vi "L2.vi"() -> ()   [LabVIEW 2014]
panel:
  out "Boolean":bool
  in  "LIMITARE":bool
  out "Tank":dbl(slide) scale=0.0..10.0 scale format="%#_2g"
  in  "MAX":dbl(slide) scale=0.0..10.0
  in  "MIN":dbl(slide) scale=0.0..10.0
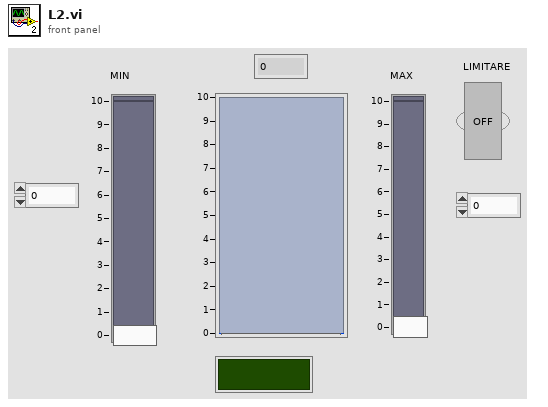
[diagram p1: front panel]
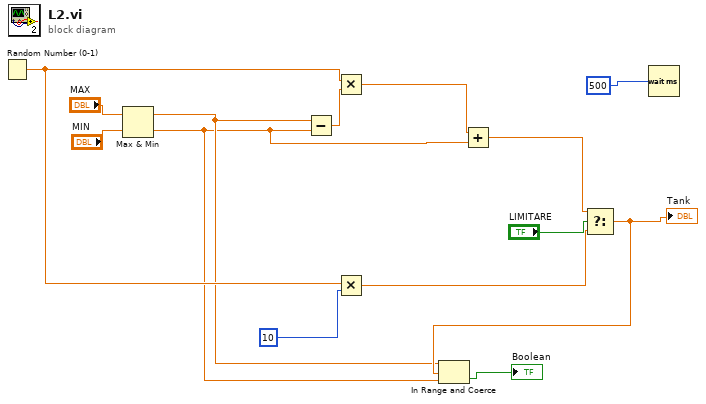
[diagram p0: block diagram]
diagram:
  n1 = Random Number (0-1)() -> (number: 0 to 1=w12:dbl)
  n2 = Max & Min(x="MAX", y="MIN") -> (max(x,y)=w2:dbl, min(x,y)=w1:dbl)
  n3 = Subtract(x=w2, y=w1) -> (x-y=w14:dbl)
  n4 = Multiply(x=w12, y=w14) -> (x*y=w13:dbl)
  n5 = Multiply(x=w12, y=10) -> (x*y=w8:dbl)
  n6 = Add(x=w13, y=w1) -> (x+y=w9:dbl)
  n7 = Select(t=w9, s="LIMITARE", f=w8) -> (s? t:f=w7:dbl)
  "Tank" <- w7
  n8 = In Range and Coerce(upper limit=w2, x=w7, lower limit=w1) -> (In Range?=→"Boolean":bool)  [unwired: 1 out]
  n9 = Wait (ms)(milliseconds to wait=500) -> ()  [unwired: 1 out]
